vi "Run Tests.vi"() -> ()   [LabVIEW 2019]
uses:
  Typedefs/Generation options.ctl
  Typedefs/Tab.ctl
panel:
  out "Passed?":T1(array[cluster])
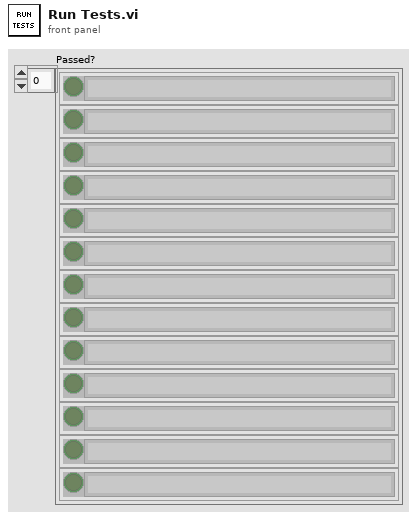
[diagram p1: front panel]
types:
  T1 = cluster{bool, "filename without extension":string}[]
  T2 = typedef "Generation options.ctl" = cluster{"Minify?":bool, "Disabled Tabs":T3[], "Default Tab":T3}
  T3 = typedef "Tab.ctl" = enum16{"Info", "FP", "BD"}
  T4 = cluster{bool, "filename without extension":string}
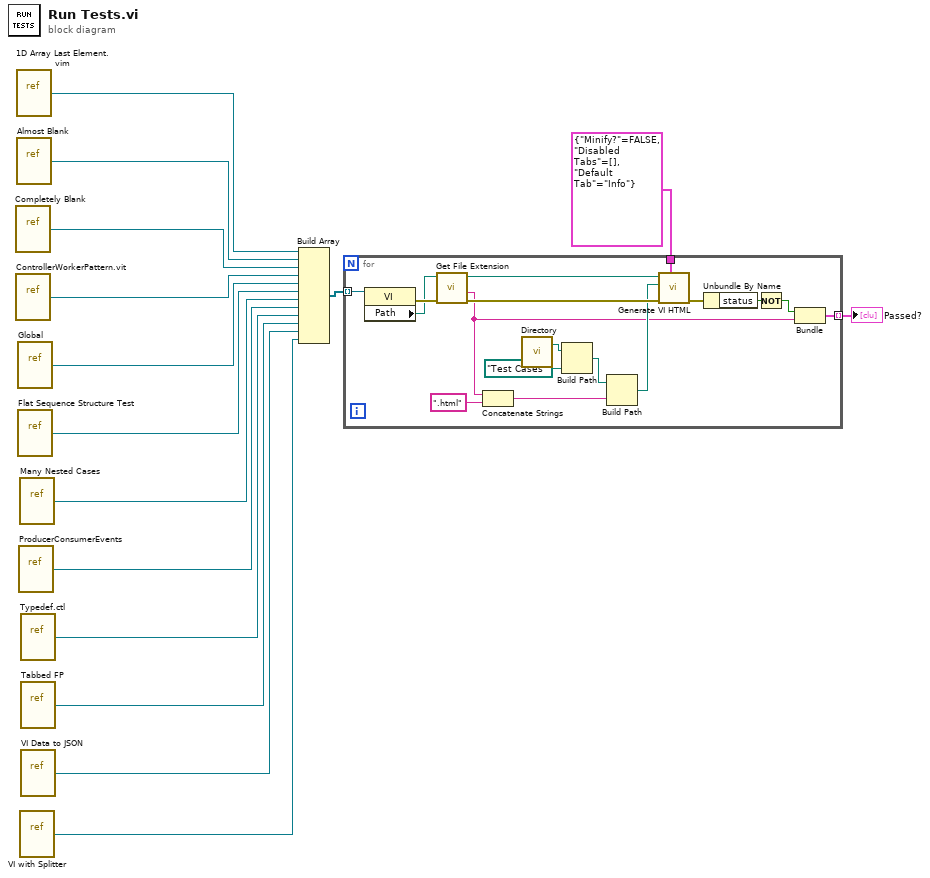
[diagram p0: block diagram]
diagram:
  n1 = vi-ref "Completely Blank.vi"() -> (w14:refnum<vi>)
  n2 = vi-ref "ControllerWorkerPattern.vit"() -> (w13:refnum<vi>)
  n3 = vi-ref "1D Array Last Element.vim"() -> (w7:refnum<vi>)
  n4 = vi-ref "Almost Blank.vi"() -> (w15:refnum<vi>)
  n5 = vi-ref "Global.vi"() -> (w12:refnum<vi>)
  n6 = vi-ref "Flat Sequence Structure Test.vi"() -> (w4:refnum<vi>)
  n7 = vi-ref "ProducerConsumerEvents.vi"() -> (w11:refnum<vi>)
  n8 = vi-ref "Many Nested Cases.vi"() -> (w8:refnum<vi>)
  n9 = vi-ref "VI with Splitter.vi"() -> (w1:refnum<vi>)
  n10 = vi-ref "Typedef.ctl"() -> (w9:refnum<vi>)
  n11 = vi-ref "Tabbed FP.vi"() -> (w2:refnum<vi>)
  n12 = vi-ref "VI Data to JSON.vi"() -> (w6:refnum<vi>)
  n13 = Build Array(w7, w15, w14, w13, w12, w4, w8, w11, w9, w2, w6, w1) -> (w10:refnum<vi>[])
  n14 = for {
    tunnel: w10 -> [w32] mode=indexing
    tunnel: T2 {"Minify?"=FALSE, "Disabled Tabs"=[], "Default Tab"=enum."Info"} ("Generation options") -> [w19]
    tunnel: [w16] -> w3 mode=indexing
    n15 = property class="VI"(reference=w32) -> (error out=w31:errorcluster, "Path"=w28:path)  [unwired: 1 in, 1 out]
    n16 = call <vilib>:"Get File Extension.vi"("error in (no error)"=w31, "file"=w28) -> ("error out"=w30:errorcluster, "filename without extension"=w17:string, "dup file"=w29:path)  [unwired: 5 in, 2 out]
    n17 = Concatenate Strings(w17, ".html" ("string")) -> (w26:string)
    n18 = call "Directory.vi"() -> ("Directory"=w22:path)  [unwired: 3 in]
    n19 = Build Path(base path=w22, name or relative path=path "Test Cases") -> (appended path=w20:path)
    n20 = Build Path(base path=w20, name or relative path=w26) -> (appended path=w25:path)
    n21 = call "Generate VI HTML.vi"("Generation options"=w19, "error in"=w30, "Output path"=w25, "VI Path"=w29) -> ("error out"=w23:errorcluster)  [unwired: 7 in]
    n22 = Unbundle By Name(w23) -> ("status"=w24:bool)
    n23 = Not(x=w24) -> (.not. x?=w18:bool)
    n24 = Bundle(w18, "filename without extension"=w17) -> (w16:T4)  [unwired: 1 in]
  }
  "Passed?" <- w3
